vi "扩展ASCII表.vi"() -> ()   [LabVIEW 2012]
panel:
  out "ASCII（224-255）":string[][](table)
  out "ASCII（192-223）":string[][](table)
  out "ASCII（160-191）":string[][](table)
  out "ASCII（128-159）":string[][](table)
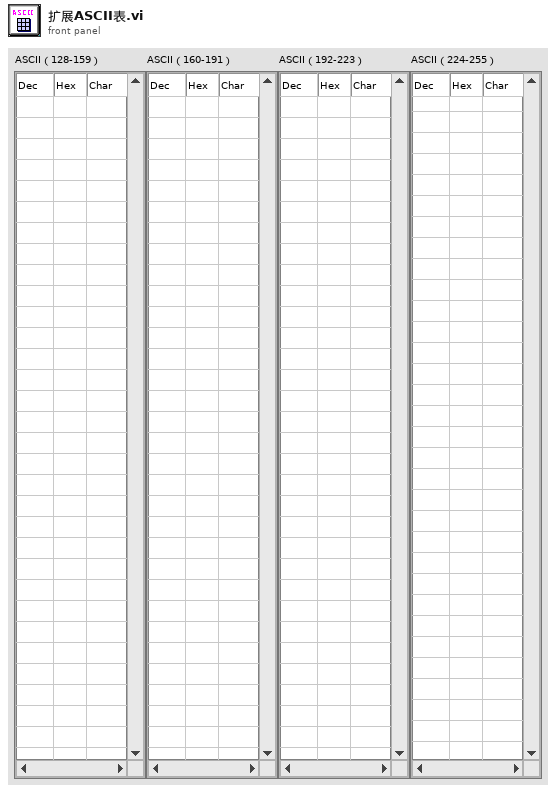
[diagram p1: front panel]
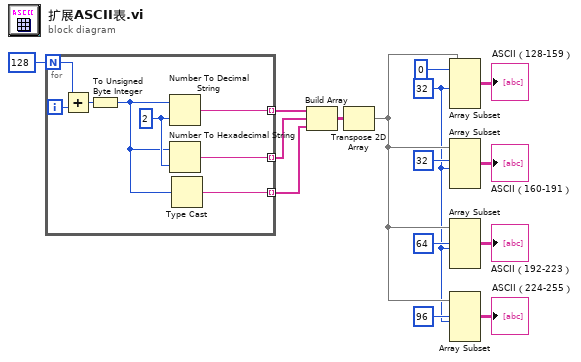
[diagram p0: block diagram]
diagram:
  w1 = 32 ("索引")
  n1 = for {
    N: 128 -> [w16]
    tunnel: [w23] -> w14 mode=indexing
    tunnel: [w22] -> w13 mode=indexing
    tunnel: [w21] -> w12 mode=indexing
    i -> [w19]
    w20 = i16 2 ("宽度(-)")
    n2 = Add(x=w16, y=w19) -> (x+y=w18:i32)
    n3 = To Unsigned Byte Integer(number=w18) -> (unsigned 8bit integer=w17:u8)
    n4 = Number To Decimal String(number=w17, width (-)=w20) -> (decimal integer string=w23:string)
    n5 = Number To Hexadecimal String(1:w20, 2:w17) -> (0:w22:string)
    n6 = Type Cast(x=w17) -> (*(type *) &x=w21:string)  [unwired: 1 in]
  }
  n7 = Build Array(w14, w13, w12) -> (w6:string[][])
  n8 = Transpose 2D Array(2D array=w6) -> (transposed array=w2:string[][])
  n9 = Array Subset(array=w2, index (row)=0 ("索引"), length (row)=w1) -> (→"ASCII（128-159）":string[][])  [unwired: 2 in]
  n10 = Array Subset(array=w2, index (row)=32 ("索引"), length (row)=w1) -> (→"ASCII（160-191）":string[][])  [unwired: 2 in]
  n11 = Array Subset(array=w2, index (row)=64 ("索引"), length (row)=w1) -> (→"ASCII（192-223）":string[][])  [unwired: 2 in]
  n12 = Array Subset(array=w2, index (row)=96 ("索引"), length (row)=w1) -> (→"ASCII（224-255）":string[][])  [unwired: 2 in]
